vi "DB Table Read & Write.vi"(8 "error in":errorcluster={"status"=FALSE, "code"=1026, "source"="Invoke Node in General Config.vi"}, 9 "reference":refnum<vi>) -> (0 "error out":errorcluster, 1 "referenceOut":refnum<vi>)   [LabVIEW 2015]
uses:
  Control Button/Exit.ctl
  Control Button/Save.ctl
panel:
  in  "Table Control":string[][](table)
  in  "Save":T1
  in  "Exit":T2
  in  "Message Box":string
  # "LO List Modification Window"
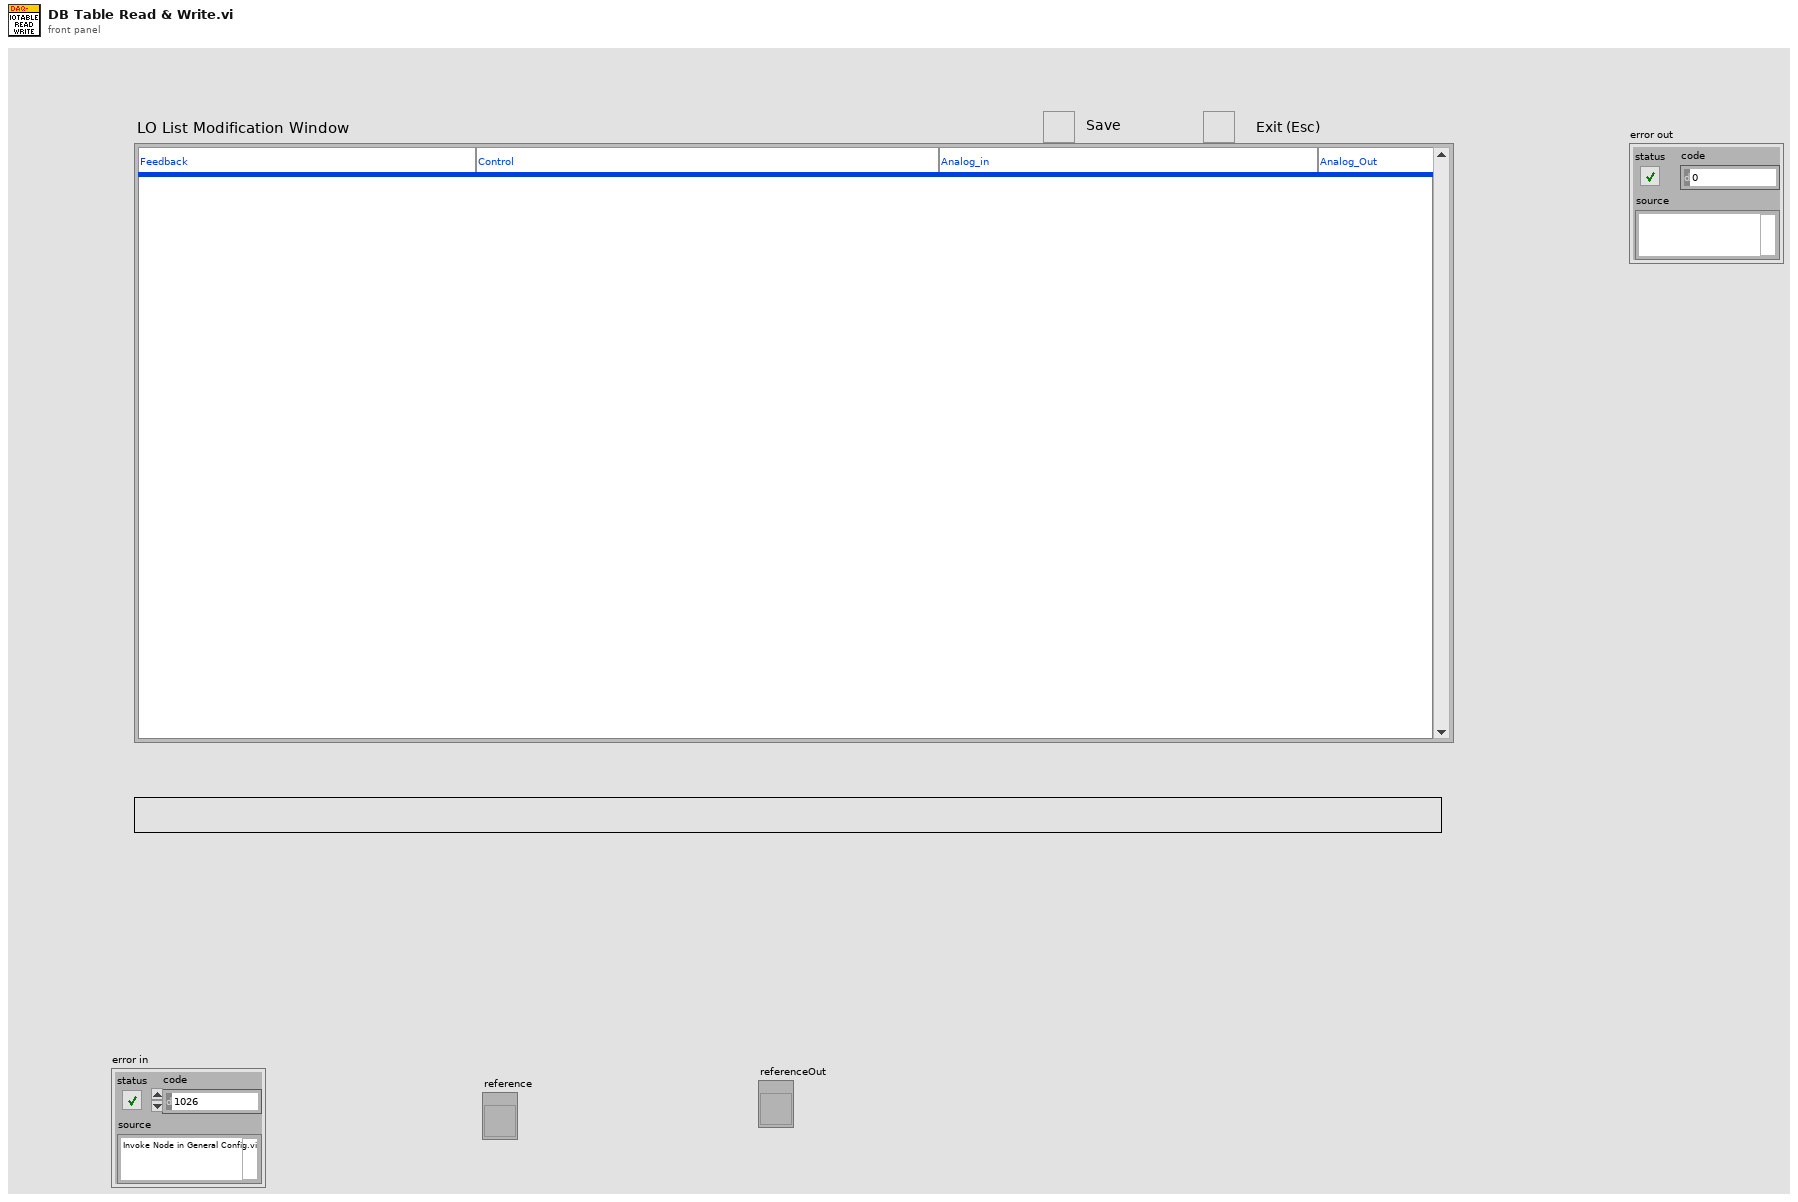
[diagram p1: front panel]
types:
  T1 = typedef "Save.ctl" = bool
  T2 = typedef "Exit.ctl" = bool
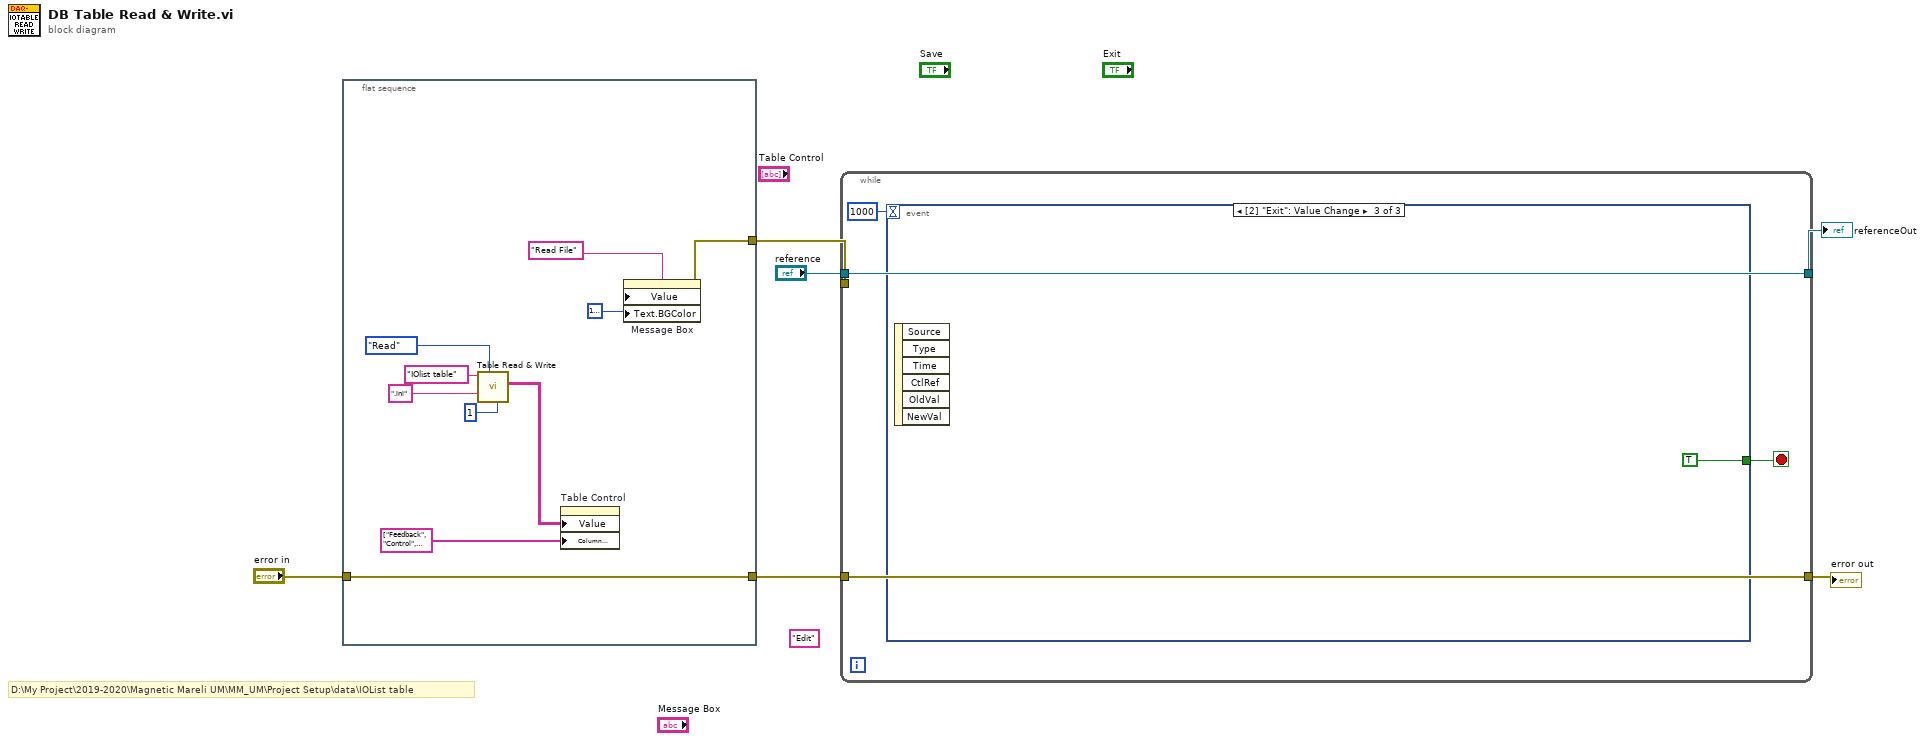
[diagram p0: block diagram]
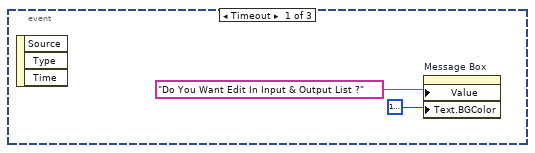
[diagram p2: hidden frame]
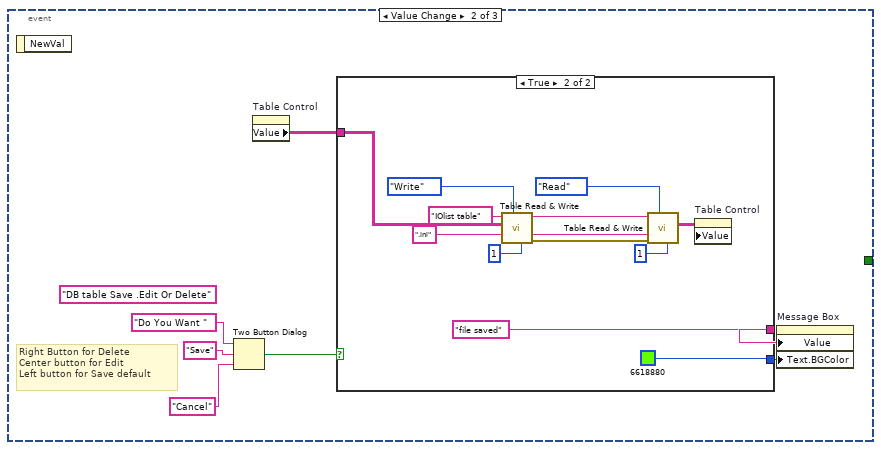
[diagram p3: hidden frame]
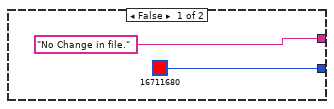
[diagram p4: hidden frame]
diagram:
  (unwired) "Edit" ("Left Button Text (\"Yes\")")
  # "D:\\My Project\\2019-2020\\Magnetic Mareli UM\\MM_UM\\Project Setup\\data\\IOList table"
  n1 = flat-sequence {
    tunnel: [w14] -> w4
    tunnel: [w15] -> w6
    tunnel: "error in" -> [w14]
    frame #0 {
      n2 = call "Table Read & Write.vi"("File Name"="IOlist table", "File type"=".ini", "Enum"=enum16{"Read", "Write"}."Read", "index"=1) -> ("Read Table"=w9:string[][])  [unwired: 5 in, 1 out]
      n3 = property on="Table Control" class="Tbl (strict)"("Value"=w9, "Column Headers[]"=string[] ["Feedback", "Control", "Analog_in", "Analog_Out"] ("Header columns")) -> ()  [unwired: 2 in, 2 out]
      n4 = property on="Message Box" class="Str"("Value"="Read File", "Text.BGColor"=u32 16777225 ("Color Box")) -> (error out=w15:errorcluster)  [unwired: 2 in, 1 out]
    }
  }
  n5 = while {
    tunnel: w6 -> [_]
    tunnel: w4 -> [w18]
    tunnel: [w18] -> w3
    tunnel: "reference" -> [w17]
    tunnel: [w17] -> w1
    stop <- w20 stop-if-true
    n6 = event shown="[2] \"Exit\": Value Change" {
      selector: _ -> [_ _ _]
      dyn-events: _ -> [_ _ _]
      timeout: 1000 -> [_ _ _]
      tunnel: [_ _ TRUE] -> w20
      event Timeout {
        n7 = event-data() -> ()  [unwired: 1 in, 3 out]
        n8 = property on="Message Box" class="Str"("Value"="Do You Want Edit In Input & Output List ?", "Text.BGColor"=u32 16777225 ("Color Box")) -> ()  [unwired: 2 in, 2 out]
      }
      event Value Change {
        (unwired) "DB table Save .Edit Or Delete" ("Window Title (\"\")")
        # "Right Button for Delete\nCenter button for Edit\nLeft button for Save default"
        n9 = event-data() -> ()  [unwired: 1 in, 1 out]
        n10 = Two Button Dialog(message="Do You Want " ("Left Button Text (\"Yes\")"), 1:"Cancel" ("Left Button Text (\"Yes\")"), 2:"Save" ("Left Button Text (\"Yes\")")) -> (T button?=w26:bool)
        n11 = property on="Table Control" class="Tbl (strict)"() -> ("Value"=w25:string[][])  [unwired: 2 in, 2 out]
        n12 = case shown="True" w26 {
          tunnel: w25 -> [_ w37]
          tunnel: ["No Change in file." ("message") "file saved" ("message")] -> w23
          tunnel: [u32 16711680 ("Color Box") u32 6618880 ("Color Box")] -> w24
          frame False {
          }
          frame True {
            w34 = ".ini" ("File type")
            w35 = "IOlist table" ("File Name")
            n13 = call "Table Read & Write.vi"("File Name"=w35, "Write Table"=w37, "File type"=w34, "Enum"=enum16{"Read", "Write"}."Write", "index"=1) -> ("error out"=w38:errorcluster)  [unwired: 4 in, 1 out]
            n14 = call "Table Read & Write.vi"("File Name"=w35, "File type"=w34, "error in"=w38, "Enum"=enum16{"Read", "Write"}."Read", "index"=1) -> ("Read Table"=w36:string[][])  [unwired: 4 in, 1 out]
            n15 = property on="Table Control" class="Tbl (strict)"("Value"=w36) -> ()  [unwired: 2 in, 2 out]
          }
        }
        n16 = property on="Message Box" class="Str"("Value"=w23, "Text.BGColor"=w24) -> ()  [unwired: 2 in, 2 out]
      }
      event Value Change {
        n17 = event-data() -> ()  [unwired: 1 in, 6 out]
      }
    }
  }
  "error out" <- w3
  "referenceOut" <- w1
